vi "Get DataColumn Ref.vi"(8 "error in (no error)":errorcluster caption="错误输入（无错误）", 11 "Data Column输入":refnum<class "Data Column.lvclass">) -> (0 "error out":errorcluster caption="错误输出", 2 "DataColumn":refnum<k24>, 3 "Data Column输出":refnum<class "Data Column.lvclass">)   [LabVIEW 2012, in "Data Grid VIEW.lvlib" / "Data Column.lvclass"]
uses:
  Data Column.lvclass
  System.Data
  Data Column.lvclass/Data Column.ctl
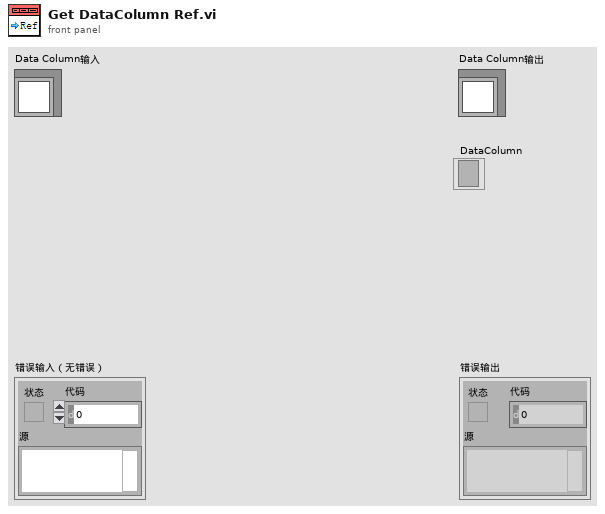
[diagram p1: front panel]
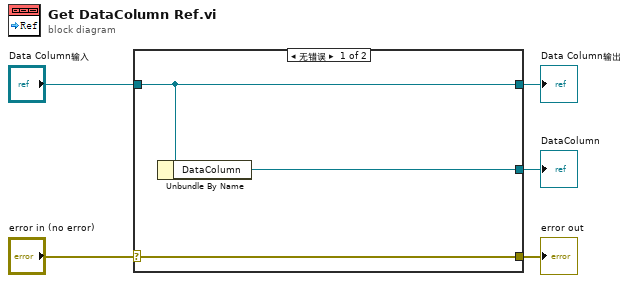
[diagram p0: block diagram]
diagram:
  n1 = case shown="无错误" "error in (no error)" {
    selector: "error in (no error)" -> [w8 w9]
    tunnel: [w8 w9] -> w4
    tunnel: [w7 w10] -> w2
    tunnel: "Data Column输入" -> [w7 w10]
    tunnel: [w6 _] -> w1
    frame No Error {
      n2 = Unbundle By Name(w7) -> ("DataColumn"=w6:refnum<k24>)
    }
    frame Error {
    }
  }
  "error out" <- w4
  "Data Column输出" <- w2
  "DataColumn" <- w1
